vi "Configure Envelope Generator.vi"(0 "Envelope Generator Handle in":refnum<k15>, 5 "Envelope Generator Configuration":T1={"Reference Clock Source"="PXI_CLK"}, 7 "Tracker Configuration":T3={"Input Impedance (Ohms)"=1000000.0, "Common Mode Offset (V)"=1.0, "Gain (V/V)"=2.5, "Output Offset (V)"=2.55} {"Input Impedance (Ohms)" format="%#_6p"}, 11 "error in":errorcluster {"code" format="%.0x"}) -> (4 "Envelope Generator Handle out":refnum<k15>, 15 "error out":errorcluster {"code" format="%.0x"})   [LabVIEW 2019, in "Envelope Tracking.lvlib"]
doc: "Configures common instrument settings for the envelope generator."
uses:
  Envelope Tracking.lvlib
  Typedefs/Tracker Configuration.ctl
  Typedefs/Envelope Generator Configuration.ctl
  <instrlib>/niRFSG/niRFSG.llb/niRFSG Ref Clock Sources.ctl
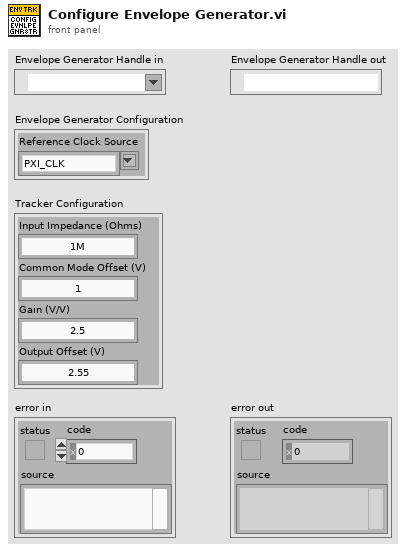
[diagram p1: front panel]
types:
  T1 = typedef "Envelope Tracking.lvlib/Envelope Generator Configuration.ctl" = cluster{"Reference Clock Source":T2}
  T2 = typedef "niRFSG Ref Clock Sources.ctl" = string
  T3 = typedef "Envelope Tracking.lvlib/Tracker Configuration.ctl" = cluster{"Input Impedance (Ohms)":dbl, "Common Mode Offset (V)":dbl, "Gain (V/V)":dbl, "Output Offset (V)":dbl}
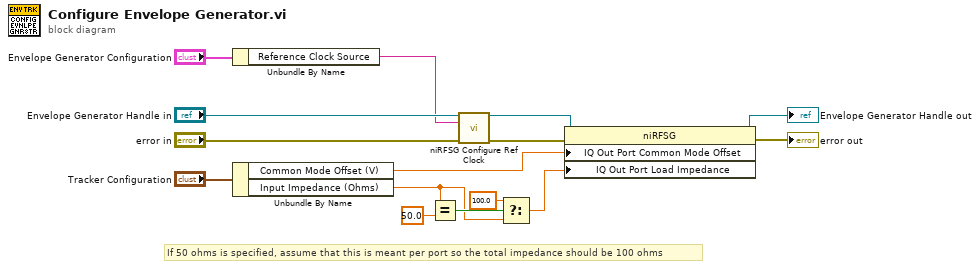
[diagram p0: block diagram]
diagram:
  # "If 50 ohms is specified, assume that this is meant per port so the total impedance should be 100 ohms"
  n1 = Unbundle By Name("Envelope Generator Configuration") -> ("Reference Clock Source"=w7:T2)
  n2 = Unbundle By Name("Tracker Configuration") -> ("Common Mode Offset (V)"=w4:dbl, "Input Impedance (Ohms)"=w6:dbl)
  n3 = Equal?(x=w6, y=50.0) -> (x = y?=w14:bool)
  n4 = call <instrlib>:"niRFSG Configure Ref Clock.vi"("instrument handle"="Envelope Generator Handle in", "ref clock source"=w7, "error in"="error in") -> ("instrument handle out"=w1:refnum<k15>, "error out"=w11:errorcluster)  [unwired: 11 in]
  n5 = Select(t=100.0 ("y"), s=w14, f=w6) -> (s? t:f=w2:dbl)
  n6 = property class="niRFSG"(reference=w1, error in=w11, "IQ Out Port Common Mode Offset"=w4, "IQ Out Port Load Impedance"=w2) -> (reference out=→"Envelope Generator Handle out":refnum<k15>, error out=→"error out":errorcluster)
